vi "Resistor Measure(NI9265).vi"(8 "error in (no error)":errorcluster caption="에러 입력(에러 없음)", 11 "열거형":enum16{"initial", "output", "stop"}(ring)) -> (0 "error out":errorcluster)   [LabVIEW 2013]
uses:
  <vilib>/DAQmx/write.llb/DAQmx Write (Analog 1D DBL NChan 1Samp).vi
  <vilib>/DAQmx/configure/timing.llb/DAQmx Timing (Sample Clock).vi
  <vilib>/DAQmx/create/channels.llb/DAQmx Create Channel (AO-Current-Basic).vi
  <vilib>/DAQmx/miscellaneous.llb/DAQmx Fill In Error Info.vi
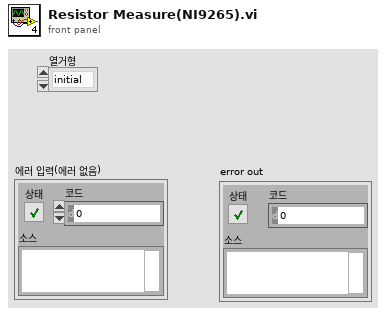
[diagram p1: front panel]
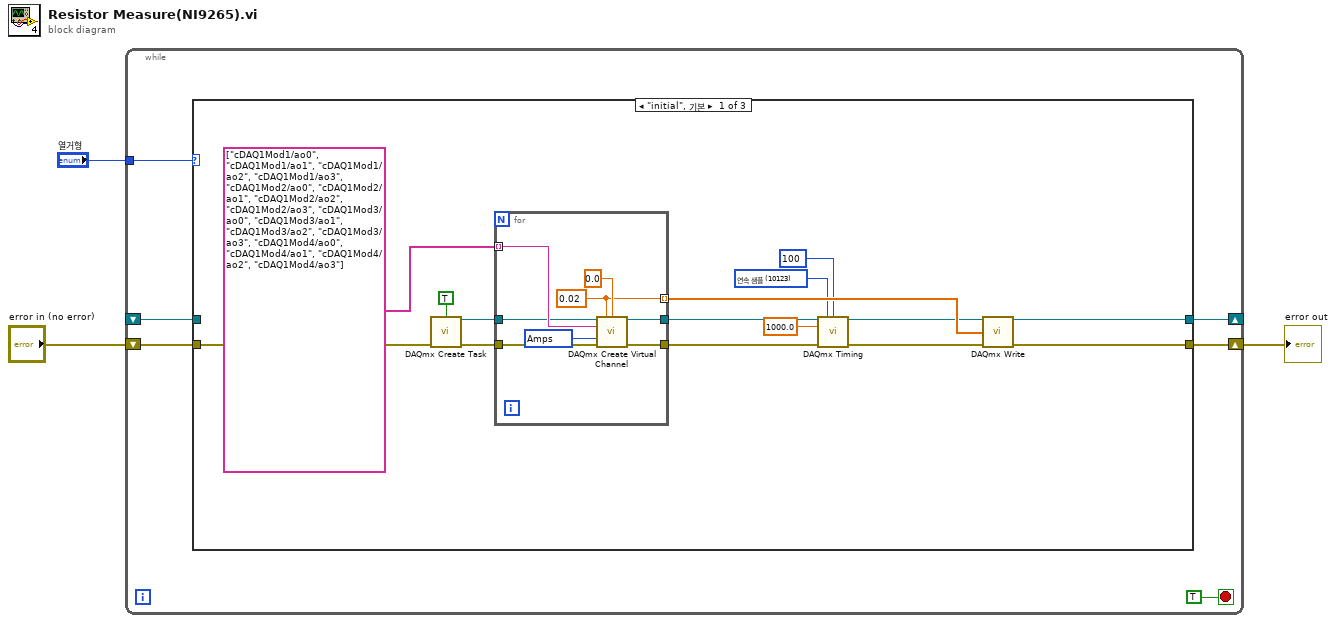
[diagram p0: block diagram]
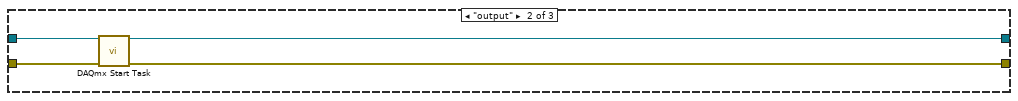
[diagram p2: hidden frame]
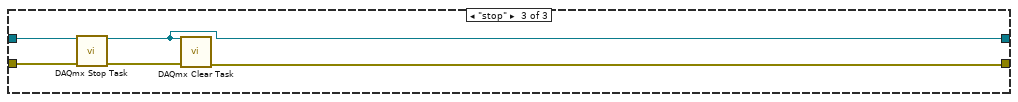
[diagram p3: hidden frame]
diagram:
  n1 = while {
    tunnel: "열거형" -> [w8]
    shift-right: [w6] -> w1
    shift-left: "error in (no error)" -> [w7]
    shift-right: [w5] -> _
    shift-left: _ -> [w4]
    stop <- TRUE stop-if-true
    n2 = case shown="\"initial\", 기본" w8 {
      tunnel: w7 -> [w20 w35 w40]
      tunnel: [w10 w33 w37] -> w6
      tunnel: [w11 w34 w38] -> w5
      tunnel: w4 -> [_ w36 w41]
      frame "initial", Default {
        w15 = 10123 items=["유한 샘플"=10178, "연속 샘플"=10123, "하드웨어 타이밍에 의한 단일 포인트"=12522] ("sample mode")
        n3 = call <vilib>:"DAQmx Create Task.vi"("auto cleanup"=TRUE, "error in"=w20) -> ("task out"=w22:refnum<k21>, "error out"=w21:errorcluster)  [unwired: 12 in]
        n4 = for {
          tunnel: tag[] ["cDAQ1Mod1/ao0", "cDAQ1Mod1/ao1", "cDAQ1Mod1/ao2", "cDAQ1Mod1/ao3", "cDAQ1Mod2/ao0", "cDAQ1Mod2/ao1", "cDAQ1Mod2/ao2", "cDAQ1Mod2/ao3", "cDAQ1Mod3/ao0", "cDAQ1Mod3/ao1", "cDAQ1Mod3/ao2", "cDAQ1Mod3/ao3", "cDAQ1Mod4/ao0", "cDAQ1Mod4/ao1", "cDAQ1Mod4/ao2", "cDAQ1Mod4/ao3"] -> [w30] mode=indexing
          tunnel: [w29] -> w18
          tunnel: [w28] -> w17
          tunnel: w22 -> [w27]
          tunnel: w21 -> [w26]
          tunnel: [w25] -> w19 mode=indexing
          w25 = 0.02 ("maximum value")
          w31 = 10342 items=["Amps"=10342, "사용자 스케일로부터"=10065] ("units")
          n5 = call-poly <vilib>:"DAQmx Create Virtual Channel.vi"("task in"=w27, "maximum value"=w25, "minimum value"=0.0, "physical channels"=w30, "units"=w31, "error in"=w26) -> ("task out"=w29:refnum<k21>, "error out"=w28:errorcluster)  [unwired: 8 in]
        }
        n6 = call-poly <vilib>:"DAQmx Timing.vi"("task/channels in"=w18, "sample mode"=w15, "samples per channel"=100, "rate"=1000.0, "error in"=w17) -> ("task out"=w13:refnum<k21>, "error out"=w12:errorcluster)  [unwired: 9 in]
        n7 = call-poly <vilib>:"DAQmx Write.vi"("task/channels in"=w13, "data"=w19, "error in"=w12) -> ("task out"=w11:refnum<k21>, "error out"=w10:errorcluster)  [unwired: 10 in, 1 out]
      }
      frame "output" {
        n8 = call <vilib>:"DAQmx Start Task.vi"("task/channels in"=w36, "error in"=w35) -> ("task out"=w34:refnum<k21>, "error out"=w33:errorcluster)  [unwired: 12 in]
      }
      frame "stop" {
        n9 = call <vilib>:"DAQmx Stop Task.vi"("task/channels in"=w41, "error in"=w40) -> ("task out"=w38:refnum<k21>, "error out"=w39:errorcluster)  [unwired: 12 in]
        n10 = call <vilib>:"DAQmx Clear Task.vi"("task in"=w38, "error in"=w39) -> ("error out"=w37:errorcluster)  [unwired: 13 in]
      }
    }
  }
  "error out" <- w1
